vi "Set Voltage and Dimming.vi"(8 "error in (no error)":errorcluster, 10 "Measurement Voltage":string, 11 "Measurement in":refnum<class "Measurement.lvclass">) -> (0 "error out":errorcluster, 3 "Measurement out":refnum<class "Measurement.lvclass">)   [LabVIEW 2015, in "Measurement.lvclass"]
uses:
  Measurement.lvclass
  Test Class/Test Class.lvclass
  Driver Test/Driver Test.lvclass
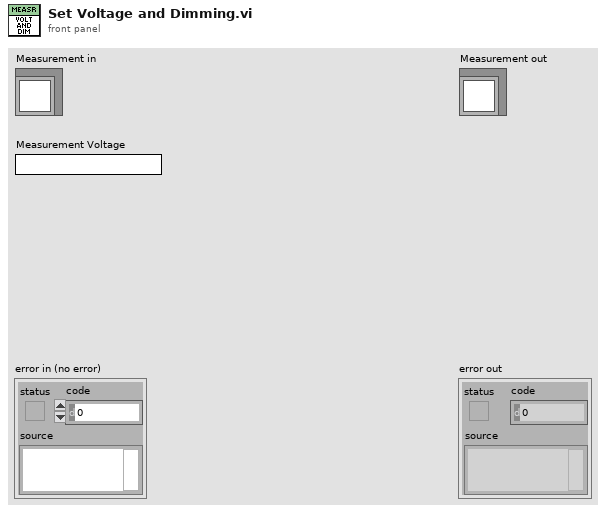
[diagram p1: front panel]
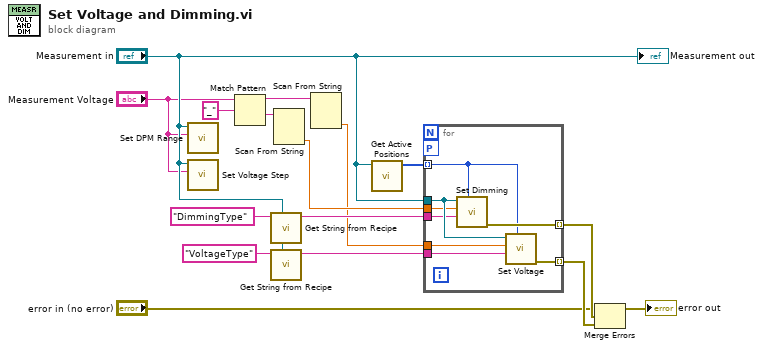
[diagram p0: block diagram]
diagram:
  n1 = call "Set DPM Range.vi"("Measurement Voltage"="Measurement Voltage", "Measurement in"="Measurement in") -> ()  [unwired: 8 in, 2 out]
  n2 = call "Set Voltage Step.vi"("Voltage Step"="Measurement Voltage", "Driver Test in"="Measurement in") -> ()  [unwired: 9 in, 1 out]
  n3 = Match Pattern(string="Measurement Voltage", regular expression="_") -> (before substring=w10:string, after substring=w11:string)  [unwired: 1 in, 2 out]
  n4 = call "Get String from Recipe.vi"("Test Class in"="Measurement in", "Name"="DimmingType") -> ("Value"=w6:string)  [unwired: 7 in, 2 out]
  n5 = call "Get String from Recipe.vi"("Test Class in"="Measurement in", "Name"="VoltageType") -> ("Value"=w7:string)  [unwired: 7 in, 2 out]
  n6 = Scan From String(input string=w11) -> (output 1=w5:dbl)  [unwired: 4 in, 3 out]
  n7 = Scan From String(input string=w10) -> (output 1=w4:dbl)  [unwired: 4 in, 3 out]
  n8 = call "Get Active Positions.vi"("Test Class in"="Measurement in") -> ("Active Positions"=w3:u32[])  [unwired: 9 in, 1 out]
  n9 = for {
    tunnel: [w23] -> w16 mode=indexing
    tunnel: [w22] -> w15 mode=indexing
    tunnel: w7 -> [w21]
    tunnel: w6 -> [w20]
    tunnel: w5 -> [w19]
    tunnel: w4 -> [w17]
    tunnel: "Measurement in" -> [w24]
    workers-P: _ -> [_]
    tunnel: w3 -> [w18] mode=indexing
    n10 = call "Set Dimming.vi"("Position"=w18, "Dimming Type"=w20, "Dim Level"=w19, "Driver Test in"=w24) -> ("error out"=w23:errorcluster)  [unwired: 7 in]
    n11 = call "Set Voltage.vi"("Position"=w18, "Voltage Type"=w21, "Voltage"=w17, "Driver Test in"=w24) -> ("error out"=w22:errorcluster)  [unwired: 7 in]
  }
  n12 = Merge Errors("error in (no error)", w16, w15) -> (→"error out":errorcluster)
  "Measurement out" <- "Measurement in"
